vi "IPI_StringChangeOption.vi"(11 "Input String":string) -> (3 "输出簇":T3 {"Edge Options"."Edge Polarity" items=["All Edges", "Rising Edges", "Falling Edges"]; "Edge Options"."Minimum Edge Strength" format="%.2f"; "Edge Options"."Width" step=2; "Edge Options"."Kernel Size" step=2})   [LabVIEW 2015]
uses:
  <vilib>/vision/Measure.llb/Edge Options.ctl
  <vilib>/vision/Measure.llb/Edge Polarity.ctl
panel:
  out "数组":string[](array[string])
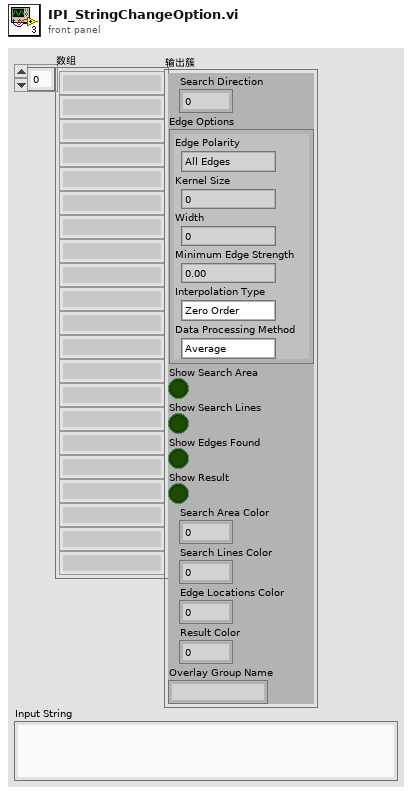
[diagram p1: front panel]
types:
  T1 = typedef "Edge Options.ctl" = cluster{"Edge Polarity":T2, "Kernel Size":u32, "Width":u32, "Minimum Edge Strength":sgl, "Interpolation Type":enum32{"Zero Order", "Bilinear", "Quadratic", "Cubic", "Bilinear Fixed"}, "Data Processing Method":enum32{"Average", "Median"}}
  T2 = typedef "Edge Polarity.ctl" = u32
  T3 = cluster{"Search Direction":u32, "Edge Options":T1, "Show Search Area":bool, "Show Search Lines":bool, "Show Edges Found":bool, "Show Result":bool, "Search Area Color":u32, "Search Lines Color":u32, "Edge Locations Color":u32, "Result Color":u32, "Overlay Group Name":string}
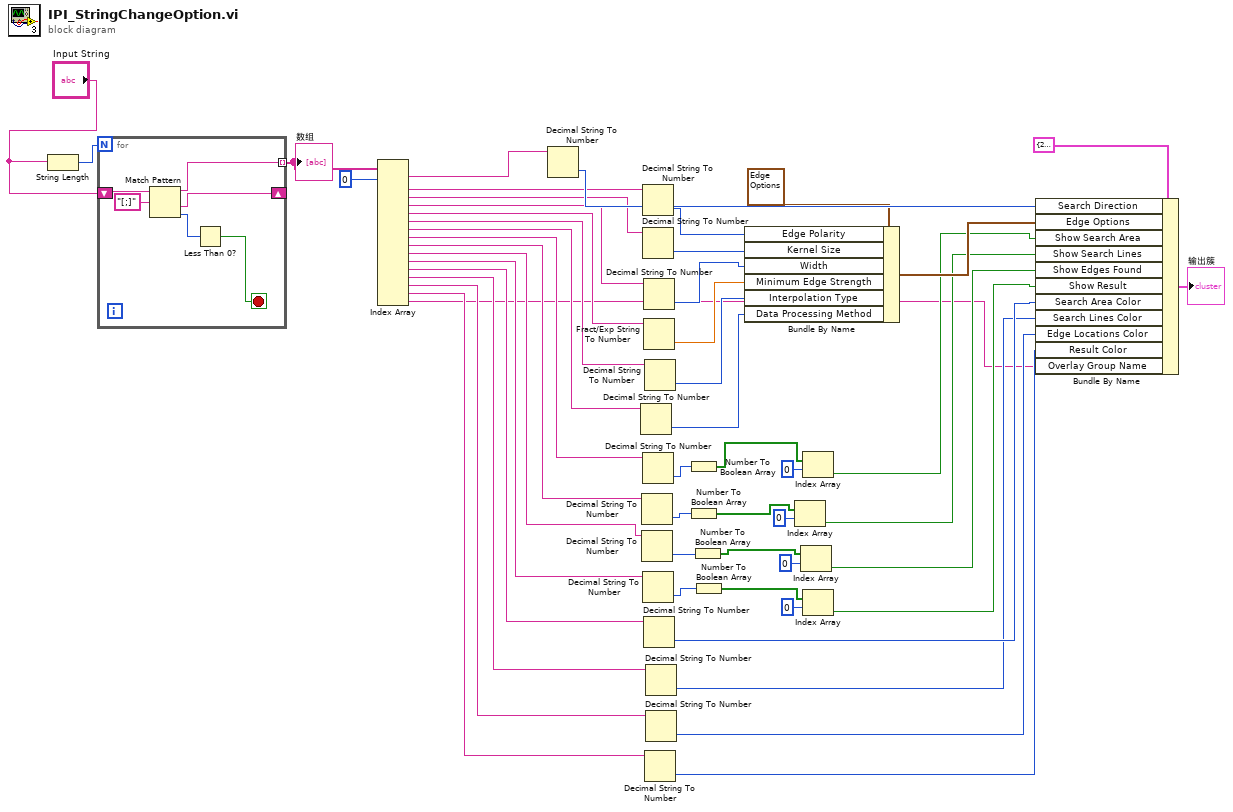
[diagram p0: block diagram]
diagram:
  n1 = String Length(string="Input String") -> (length=w51:i32)
  n2 = for {
    N: w51 -> [_]
    shift-right: [w56] -> _
    shift-left: "Input String" -> [w57]
    tunnel: [w54] -> w49 mode=indexing
    stop <- w52 stop-if-true
    n3 = Match Pattern(string=w57, regular expression="[;]" ("正则表达式")) -> (before substring=w54:string, after substring=w56:string, offset past match=w53:i32)  [unwired: 1 in, 1 out]
    n4 = Less Than 0?(x=w53) -> (x < 0?=w52:bool)
  }
  "数组" <- w49
  n5 = Index Array(array=w49, index #1=0 ("索引")) -> (element #1=w47:string, element #2=w45:string, element #3=w44:string, element #4=w43:string, element #5=w42:string, element #6=w41:string, element #7=w40:string, element #8=w31:string, element #9=w30:string, element #10=w29:string, element #11=w28:string, element #12=w11:string, element #13=w10:string, element #14=w9:string, element #15=w8:string, element #16=w3:string)  [unwired: 15 in]
  n6 = Decimal String To Number(string=w47) -> (number=w46:i32)  [unwired: 2 in, 1 out]
  n7 = Decimal String To Number(string=w40) -> (number=w33:i32)  [unwired: 2 in, 1 out]
  n8 = Decimal String To Number(string=w30) -> (number=w26:i32)  [unwired: 2 in, 1 out]
  n9 = Decimal String To Number(string=w29) -> (number=w25:i32)  [unwired: 2 in, 1 out]
  n10 = Decimal String To Number(string=w45) -> (number=w38:i32)  [unwired: 2 in, 1 out]
  n11 = Decimal String To Number(string=w44) -> (number=w37:i32)  [unwired: 2 in, 1 out]
  n12 = Decimal String To Number(string=w31) -> (number=w27:i32)  [unwired: 2 in, 1 out]
  n13 = Decimal String To Number(string=w28) -> (number=w24:i32)  [unwired: 2 in, 1 out]
  n14 = Decimal String To Number(string=w43) -> (number=w36:i32)  [unwired: 2 in, 1 out]
  n15 = Fract/Exp String To Number(string=w42) -> (number=w35:dbl)  [unwired: 3 in, 1 out]
  n16 = Decimal String To Number(string=w11) -> (number=w7:i32)  [unwired: 2 in, 1 out]
  n17 = Decimal String To Number(string=w41) -> (number=w34:i32)  [unwired: 2 in, 1 out]
  n18 = Decimal String To Number(string=w8) -> (number=w4:i32)  [unwired: 2 in, 1 out]
  n19 = Decimal String To Number(string=w10) -> (number=w6:i32)  [unwired: 2 in, 1 out]
  n20 = Decimal String To Number(string=w9) -> (number=w5:i32)  [unwired: 2 in, 1 out]
  n21 = Number To Boolean Array(number=w27) -> (Boolean array=w23:bool[])
  n22 = Number To Boolean Array(number=w26) -> (Boolean array=w18:bool[])
  n23 = Number To Boolean Array(number=w25) -> (Boolean array=w17:bool[])
  n24 = Number To Boolean Array(number=w24) -> (Boolean array=w16:bool[])
  n25 = Bundle By Name(cluster=T1 {"Edge Polarity"=0, "Kernel Size"=3, "Width"=3, "Minimum Edge Strength"=10.0, "Interpolation Type"=enum."Bilinear Fixed", "Data Processing Method"=enum."Average"} ("Edge Options 2"), "Edge Polarity"=w38, "Kernel Size"=w37, "Width"=w36, "Minimum Edge Strength"=w35, "Interpolation Type"=w34, "Data Processing Method"=w33) -> (w32:T1)
  n26 = Index Array(array=w18, index=0 ("索引")) -> (element=w14:bool)
  n27 = Index Array(array=w17, index=0 ("索引")) -> (element=w13:bool)
  n28 = Index Array(array=w23, index=0 ("索引")) -> (element=w15:bool)
  n29 = Index Array(array=w16, index=0 ("索引")) -> (element=w12:bool)
  n30 = Bundle By Name(cluster=T3 {"Search Direction"=2, "Edge Options"={"Edge Polarity"=1, "Kernel Size"=3, "Width"=1, "Minimum Edge Strength"=21.0, "Interpolation Type"=enum."Bilinear Fixed", "Data Processing Method"=enum."Average"}, "Show Search Area"=TRUE, "Show Search Lines"=FALSE, "Show Edges Found"=FALSE, "Show Result"=TRUE, "Search Area Color"=65280, "Search Lines Color"=255, "Edge Locations Color"=16776960, "Result Color"=16711680, "Overlay Group Name"=""} ("Options (Find Straight Edge 2) 2"), "Search Direction"=w46, "Edge Options"=w32, "Show Search Area"=w15, "Show Search Lines"=w14, "Show Edges Found"=w13, "Show Result"=w12, "Search Area Color"=w7, "Search Lines Color"=w6, "Edge Locations Color"=w5, "Result Color"=w4, "Overlay Group Name"=w3) -> (→"输出簇":T3)
